vi "Refresh Listbox Changes.vi"(8 "error in":errorcluster, 9 "number of visible rows":u32, 10 "only show changes (T)":bool=TRUE, 11 "refresh listbox":T1[](array[typedef])) -> (0 "error out":errorcluster, 1 "background colors":u32[][](array[colorbox]), 2 "item symbols":T2[](array[typedef])=[enum."Blank", enum."Incoming", enum."Outgoing", enum."Label", enum."Word", enum."Parameter"], 3 "item names":string[][](array[string]))   [LabVIEW 2020, in "AIM ARINC 429 System Explorer.lvlib" / "Implementation.lvlib"]
doc: "This VI runs when the Add Port run-time menu is chosen. It allows the user to create a port with an associated database."
uses:
  Implementation.lvlib
  Types/Refresh Symbols.ctl
  Types/Refresh Listbox.ctl
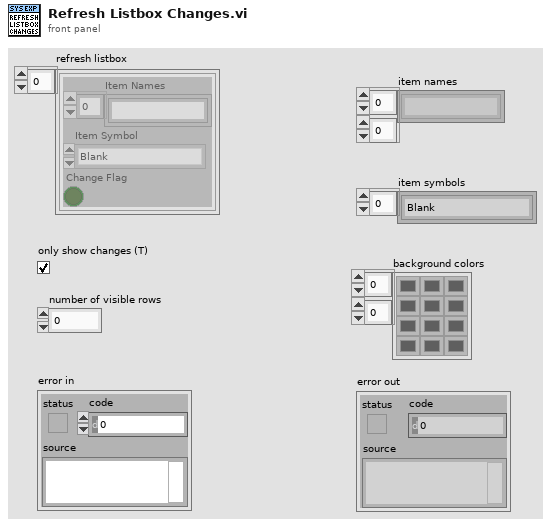
[diagram p1: front panel]
types:
  T1 = typedef "AIM ARINC 429 System Explorer.lvlib/Implementation.lvlib/Refresh Listbox.ctl" = cluster{"Item Names":string[], "Item Symbol":T2, "Change Flag":bool}
  T2 = typedef "AIM ARINC 429 System Explorer.lvlib/Implementation.lvlib/Refresh Symbols.ctl" = enum16{"Blank", "Port", "Incoming", "Outgoing", "Label", "Word", "Parameter", "ARINC-429", "Config Files", "Channel Spec", "Item"}
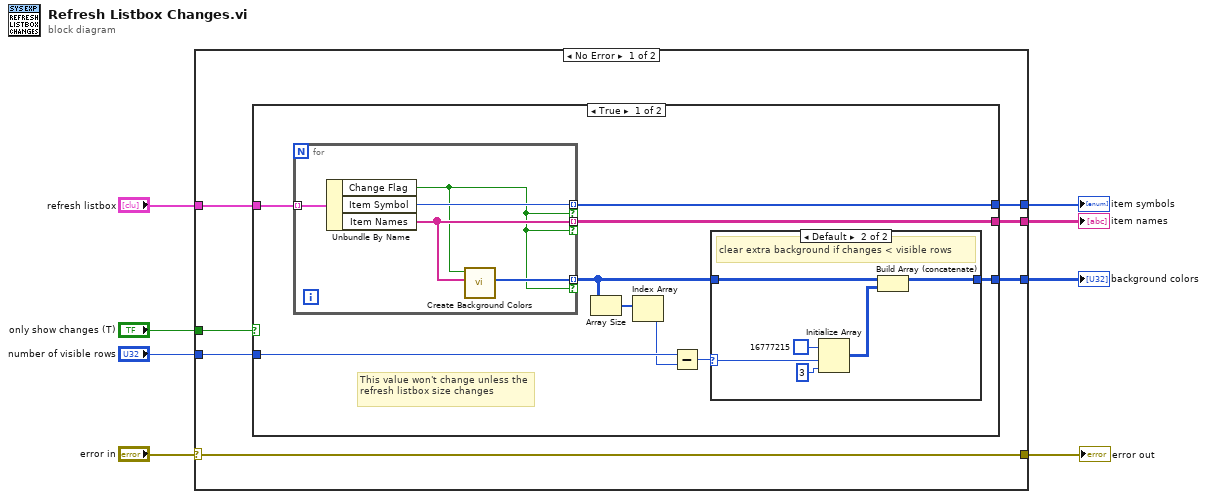
[diagram p0: block diagram]
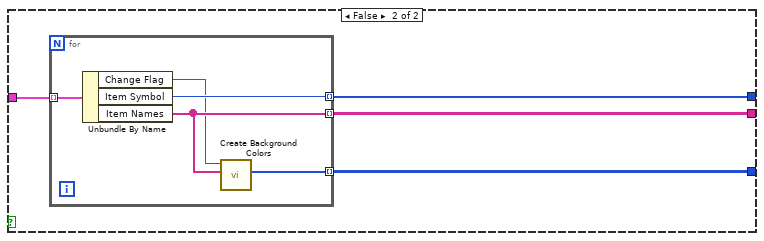
[diagram p3: hidden frame]
diagram:
  n1 = case shown="No Error" "error in" {
    selector: "error in" -> [w12 w46]
    tunnel: "refresh listbox" -> [w11 _]
    tunnel: "only show changes (T)" -> [w15 _]
    tunnel: [w14 _] -> w4
    tunnel: [w13 _] -> w3
    tunnel: [w12 w46] -> w6
    tunnel: [w10 _] -> w2
    tunnel: "number of visible rows" -> [w9 _]
    frame No Error {
      n2 = case shown="True" w15 {
        tunnel: [w24 w40] -> w14
        tunnel: [w23 w39] -> w13
        tunnel: w11 -> [w22 w38]
        tunnel: [w16 w37] -> w10
        tunnel: w9 -> [w19 _]
        frame True {
          # "This value won't change unless the refresh listbox size changes"
          n3 = for {
            tunnel: [w36] -> w24 mode=indexing if=w32
            tunnel: [w33] -> w23 mode=indexing if=w32
            tunnel: w22 -> [w35] mode=indexing
            tunnel: [w34] -> w17 mode=indexing if=w32
            n4 = Unbundle By Name(w35) -> ("Change Flag"=w32:bool, "Item Symbol"=w36:T2, "Item Names"=w33:string[])
            n5 = call "Create Background Colors.vi"("iItem names"=w33, "change flag"=w32) -> ("background colors"=w34:u32[])  [unwired: 9 in]
          }
          n6 = Array Size(array=w17) -> (size(s)=w21:i32[])
          n7 = Index Array(array=w21) -> (element=w18:i32)  [unwired: 1 in]
          n8 = Subtract(x=w19, y=w18) -> (x-y=w20:u32)
          n9 = case shown="Default" w20 {
            selector: w20 -> [_ w29]
            tunnel: w17 -> [w25 w28]
            tunnel: [w25 w26] -> w16
            frame ..0 {
              # "changes >= visible rows"
            }
            frame Default {
              # "clear extra background if changes < visible rows"
              n10 = Initialize Array(u32 16777215, w29, 3 ("dimension size")) -> (w27:u32[][])
              n11 = Build Array (concatenate)(w28, w27) -> (w26:u32[][])
            }
          }
        }
        frame False {
          n12 = for {
            tunnel: [w45] -> w40 mode=indexing
            tunnel: [w42] -> w39 mode=indexing
            tunnel: w38 -> [w44] mode=indexing
            tunnel: [w43] -> w37 mode=indexing
            n13 = Unbundle By Name(w44) -> ("Change Flag"=w41:bool, "Item Symbol"=w45:T2, "Item Names"=w42:string[])
            n14 = call "Create Background Colors.vi"("iItem names"=w42, "change flag"=w41) -> ("background colors"=w43:u32[])  [unwired: 9 in]
          }
        }
      }
    }
    frame Error {
    }
  }
  "error out" <- w6
  "item names" <- w3
  "item symbols" <- w4
  "background colors" <- w2
